vi "Get_IsSaturated.vi"(8 "error in (no error)":errorcluster, 10 "Data Raw":T1(array[cluster]), 11 "Avantes in":refnum<class "Avantes.lvclass">) -> (0 "error out":errorcluster, 2 "Is Saturated?":bool, 3 "Avantes out":refnum<class "Avantes.lvclass">)   [LabVIEW 2020, in "Avantes.lvclass"]
uses:
  <instrlib>/Classes/CCD/Avantes/Avantes.lvclass
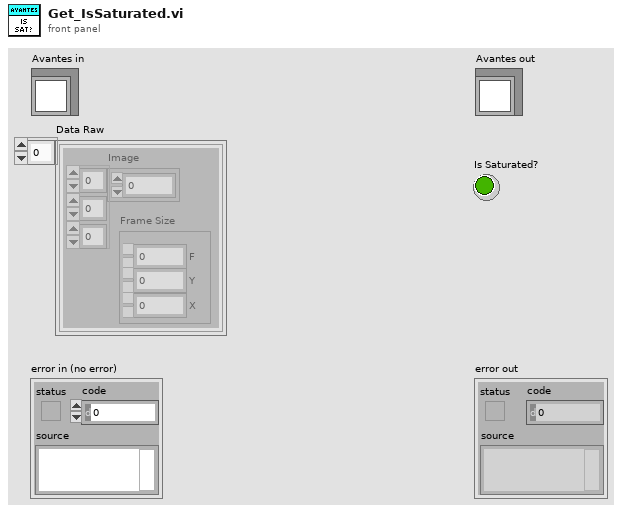
[diagram p1: front panel]
types:
  T1 = cluster{"Image":dbl[][][], "Frame Size":cluster{"F":i32, "Y":i32, "X":i32}}[]
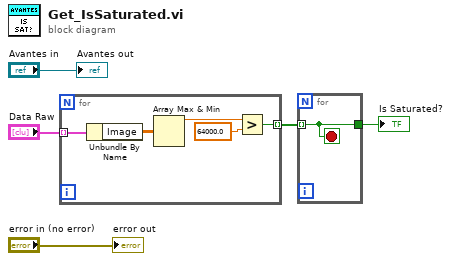
[diagram p0: block diagram]
diagram:
  n1 = for {
    tunnel: "Data Raw" -> [w10] mode=indexing
    tunnel: [w6] -> w4 mode=indexing
    n2 = Unbundle By Name(w10) -> ("Image"=w9:dbl[][][])
    n3 = Array Max & Min(array=w9) -> (max value=w8:dbl)  [unwired: 3 out]
    n4 = Greater?(x=w8, y=64000.0) -> (0:w6:bool)
  }
  n5 = for {
    tunnel: w4 -> [w11] mode=indexing
    tunnel: [w11] -> w3
    stop <- w11 stop-if-true
  }
  "Is Saturated?" <- w3
  "error out" <- "error in (no error)"
  "Avantes out" <- "Avantes in"
